vi "Parse Build Spec.vi"(0 "Export In":refnum<class "Export.lvclass">) -> (4 "Export Out":refnum<class "Export.lvclass">)   [LabVIEW 2017, in "CL_G3_VIComponentBuilder.lvlib" / "Export.lvclass"]
doc: "Parses the Export's build specification for any information required by the export."
uses:
  Export.lvclass
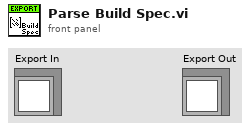
[diagram p1: front panel]
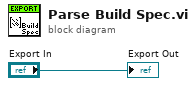
[diagram p0: block diagram]
diagram:
  "Export Out" <- "Export In"
